vi "~POC - Video Player.vi"() -> ()   [LabVIEW 2026]
uses:
  ee0876c7-fe61-481f-ab68-a2d5c60b0e47.vi
  329ef220-7369-4e64-8ff1-382a6ca25eb8.vi
  TreeDirectoryExt/TreeDirectoryExt.lvclass
  C:/Program Files/National Instruments/LabVIEW 2026/vi.lib/QSI/QControls/QControl Classes/TreeControl/TreeControl.lvclass
panel:
  in  "Table of Contents":string(tree)
  out "Web Browser Control":string(html)
  out "Run Javascript":string
  out "Exception":string
  in  "Speed":dbl(slide)=1.0 min=0.5 max=3.0 step=0.25 scale=0.5..3.0
  in  "Checkbox":bool
  in  "Stop":bool
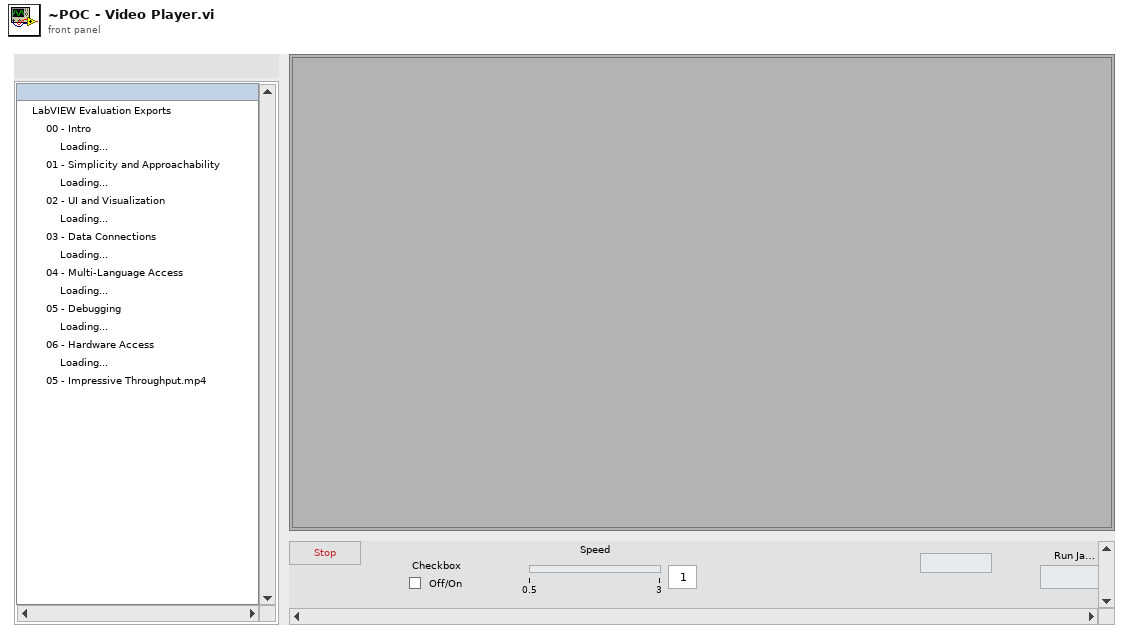
[diagram p1: front panel]
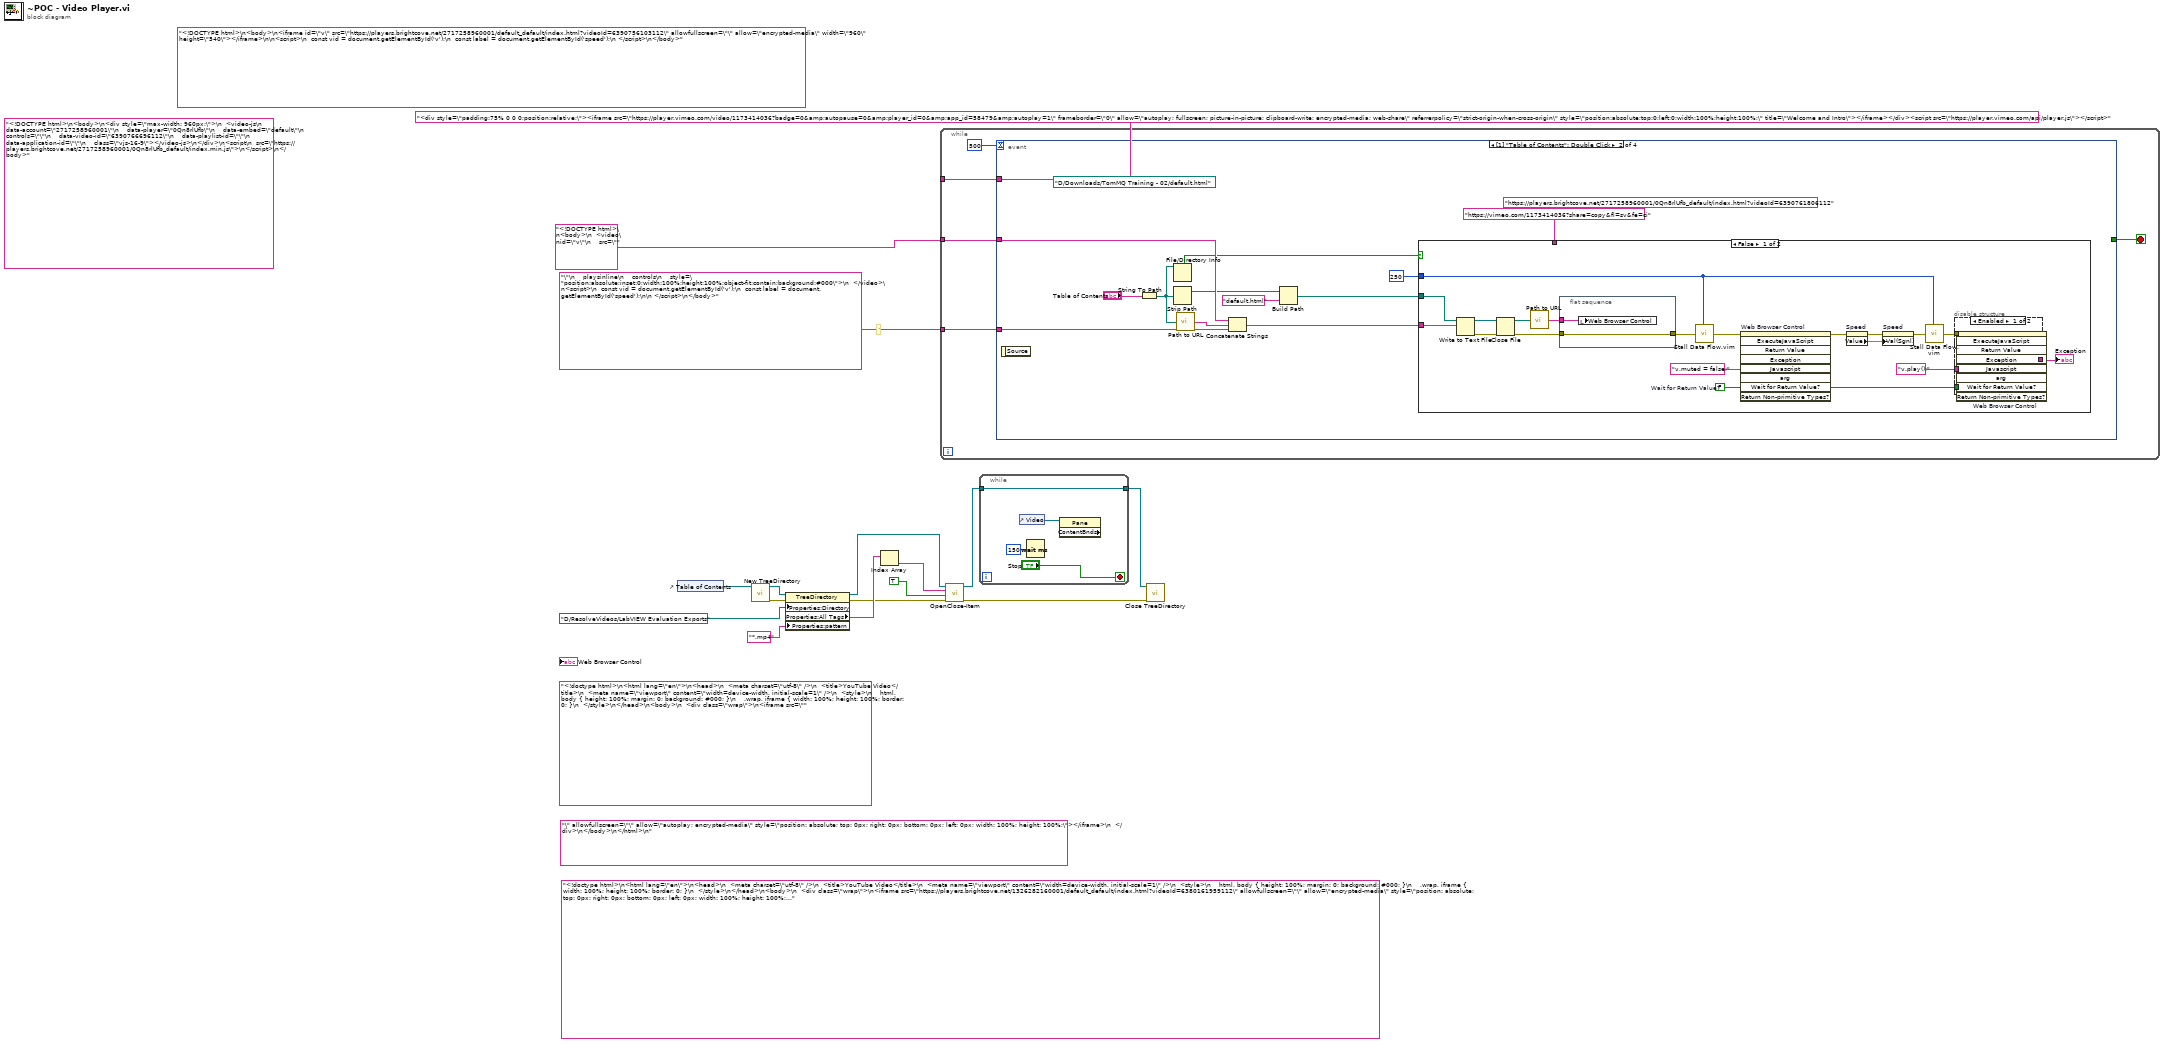
[diagram p0: block diagram]
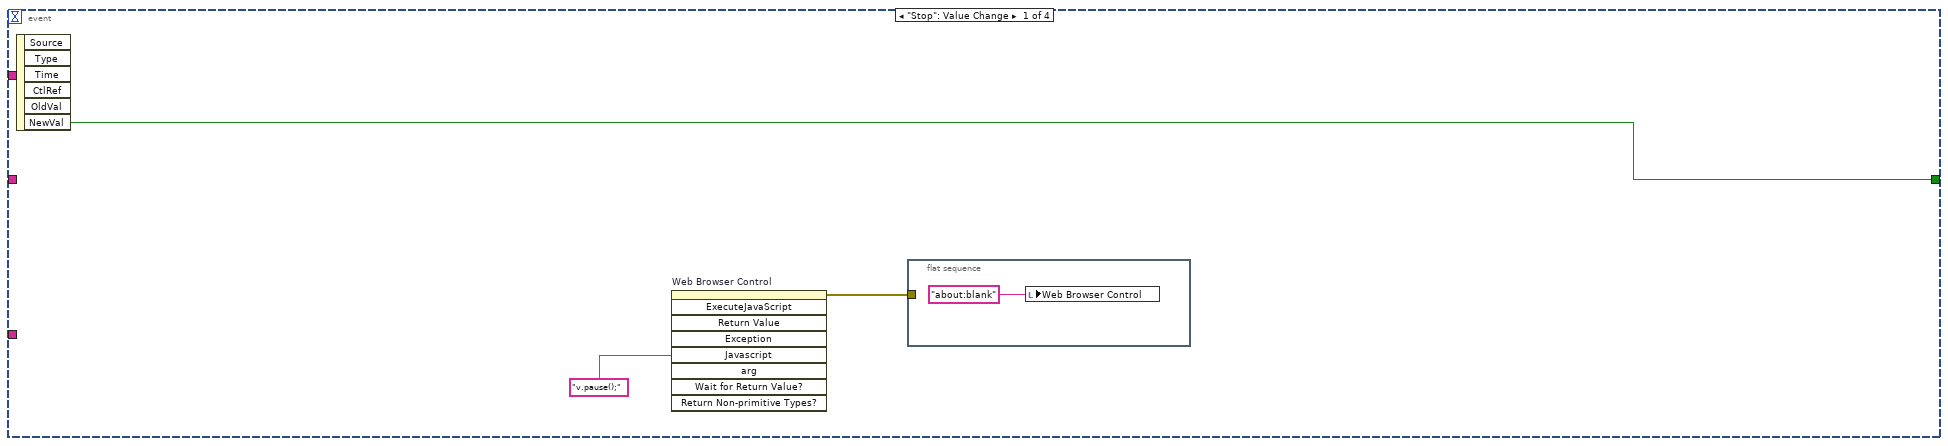
[diagram p2: hidden frame]
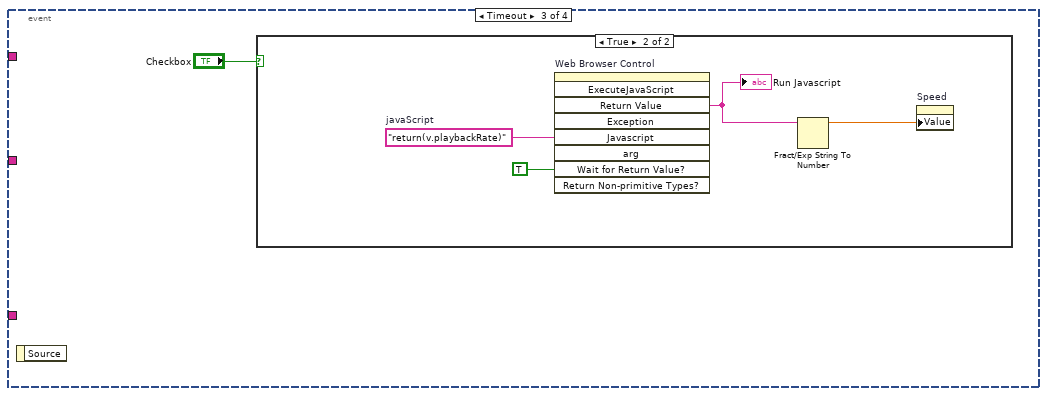
[diagram p5: hidden frame]
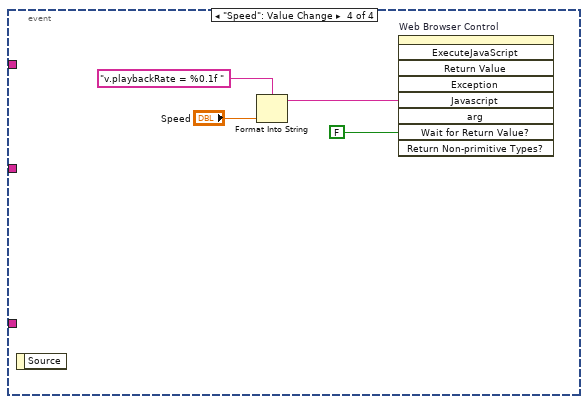
[diagram p7: hidden frame]
diagram:
  (unwired) "<!DOCTYPE html>\n<body>\n<div style=\"max-width: 960px;\">\n  <video-js\n    data-account=\"2717258960001\"\n    data-player=\"0Qn8rlUfb\"\n    data-embed=\"default\"\n    controls=\"\"\n    data-video-id=\"6390766696112\"\n    data-playlist-id=\"\"\n    data-application-id=\"\"\n    class=\"vjs-16-9\"></video-js>\n</div>\n<script\n  src=\"https://players.brightcove.net/2717258960001/0Qn8rlUfb_default/index.min.js\">\n</script>\n</body>"
  (unwired) "<!DOCTYPE html>\n<body>\n<iframe id=\"v\" src=\"https://players.brightcove.net/2717258960001/default_default/index.html?videoId=6390756103112\" allowfullscreen=\"\" allow=\"encrypted-media\" width=\"960\" height=\"540\"></iframe>\n\n<script>\n  const vid = document.getElementById('v');\n  const label = document.getElementById('speed');\n </script>\n</body>"
  (unwired) "\" allowfullscreen=\"\" allow=\"autoplay; encrypted-media\" style=\"position: absolute; top: 0px; right: 0px; bottom: 0px; left: 0px; width: 100%; height: 100%;\"></iframe>\n  </div>\n</body>\n</html>\n"
  (unwired) "<!doctype html>\n<html lang=\"en\">\n<head>\n  <meta charset=\"utf-8\" />\n  <title>YouTube Video</title>\n  <meta name=\"viewport\" content=\"width=device-width, initial-scale=1\" />\n  <style>\n    html, body { height: 100%; margin: 0; background: #000; }\n    .wrap, iframe { width: 100%; height: 100%; border: 0; }\n  </style>\n</head>\n<body>\n  <div class=\"wrap\">\n<iframe src=\"https://players.brightcove.net/1326282160001/default_default/index.html?videoId=6380161959112\" allowfullscreen=\"\" allow=\"encrypted-media\" style=\"position: absolute; top: 0px; right: 0px; bottom: 0px; left: 0px; width: 100%; height: 100%;\"></iframe>\n  </div>\n</body>\n</html>\n"
  (unwired) "<!doctype html>\n<html lang=\"en\">\n<head>\n  <meta charset=\"utf-8\" />\n  <title>YouTube Video</title>\n  <meta name=\"viewport\" content=\"width=device-width, initial-scale=1\" />\n  <style>\n    html, body { height: 100%; margin: 0; background: #000; }\n    .wrap, iframe { width: 100%; height: 100%; border: 0; }\n  </style>\n</head>\n<body>\n  <div class=\"wrap\">\n<iframe src=\""
  # "`"
  n1 = control-ref of="Table of Contents"() -> (w15:refnum<vi>)
  n2 = call "New TreeDirectory.vi"("Reference"=w15) -> ("error out"=w13:errorcluster, "TreeDirectory out"=w14:refnum<class "TreeDirectoryExt.lvclass">)  [unwired: 9 in]
  n3 = property class="TreeDirectory"(reference=w14, error in=w13, "Properties:Directory"=path "D:/ResolveVideos/LabVIEW Evaluation Exports", "Properties:pattern"="*.mp4" ("pattern")) -> (reference out=w3:refnum<class "TreeDirectoryExt.lvclass">, error out=w10:errorcluster, "Properties:All Tags"=w12:string[])
  n4 = Index Array(array=w12) -> (element=w16:string)  [unwired: 1 in]
  n5 = while {
    tunnel: "<!DOCTYPE html>\n<body>\n  <video\nid=\"v\"\n    src=\"" -> [w21]
    tunnel: "\"\n    playsinline\n    controls\n    style=\"position:absolute;inset:0;width:100%;height:100%;object-fit:contain;background:#000\">\n  </video>\n<script>\n  const vid = document.getElementById('v');\n  const label = document.getElementById('speed');\n\n </script>\n</body>" -> [w20]
    tunnel: "<div style=\"padding:75% 0 0 0;position:relative;\"><iframe src=\"https://player.vimeo.com/video/1173414036?badge=0&amp;autopause=0&amp;player_id=0&amp;app_id=58479&amp;autoplay=1\" frameborder=\"0\" allow=\"autoplay; fullscreen; picture-in-picture; clipboard-write; encrypted-media; web-share\" referrerpolicy=\"strict-origin-when-cross-origin\" style=\"position:absolute;top:0;left:0;width:100%;height:100%;\" title=\"Welcome and Intro\"></iframe></div><script src=\"https://player.vimeo.com/api/player.js\"></script>" -> [w17]
    stop <- w19 stop-if-true
    n6 = event shown="[1] \"Table of Contents\": Double Click" {
      selector: _ -> [_ _ _ _]
      dyn-events: _ -> [_ _ _ _]
      timeout: 500 -> [_ _ _ _]
      tunnel: w21 -> [_ w36 _ _]
      tunnel: w20 -> [_ w35 _ _]
      tunnel: [w24 _ _ _] -> w19
      tunnel: w17 -> [_ _ _ _]
      event "Stop": Value Change {
        n7 = event-data() -> ("NewVal"=w24:bool)  [unwired: 1 in, 5 out]
        n8 = invoke on="Web Browser Control" class="WebBrowser (strict)" method="ExecuteJavaScript"("Javascript"="v.pause();" ("javaScript")) -> (error out=w22:errorcluster)  [unwired: 8 in, 8 out]
        n9 = flat-sequence {
          tunnel: w22 -> [_]
          frame #0 {
            n10 = local write "Web Browser Control"("about:blank") -> ()
          }
        }
      }
      event "Table of Contents": Double Click {
        (unwired) "https://players.brightcove.net/2717258960001/0Qn8rlUfb_default/index.html?videoId=6390761806112"
        (unwired) path "D:/Downloads/TomMQ Training - 02/default.html"
        n11 = event-data() -> ()  [unwired: 1 in, 1 out]
        n12 = String To Path(string="Table of Contents") -> (path=w29:path)
        n13 = File/Directory Info(path=w29) -> (directory=w30:bool)  [unwired: 1 in, 6 out]
        n14 = Strip Path(path=w29) -> (stripped path=w33:path)  [unwired: 1 out]
        n15 = call <vilib>:"Path to URL.vi"("path"=w29) -> ("url"=w28:string)
        n16 = Concatenate Strings(w36, w28, w35) -> (w26:string)
        n17 = Build Path(base path=w33, name or relative path="default.html") -> (appended path=w32:path)
        n18 = case shown="False" w30 {
          tunnel: w32 -> [w56 _]
          tunnel: w26 -> [w55 _]
          tunnel: u32 250 ("milliseconds to wait") -> [w43 _]
          tunnel: "https://vimeo.com/1173414036?share=copy&fl=sv&fe=ci" -> [_ _]
          frame False {
            w42 = FALSE  # Wait for Return Value?
            n19 = Write to Text File(file (use dialog)=w56, text=w55) -> (refnum out=w53:refnum<file>, error out=w54:errorcluster)  [unwired: 2 in, 1 out]
            n20 = Close File(refnum=w53, error in=w54) -> (path=w46:path, error out=w49:errorcluster)
            n21 = call <vilib>:"Path to URL.vi"("path"=w46) -> ("url"=w38:string)
            n22 = flat-sequence {
              tunnel: [w63] -> w50
              tunnel: w49 -> [w63]
              tunnel: w38 -> [w62]
              frame #0 {
                n23 = local write "Web Browser Control"(w62) -> ()
              }
            }
            n24 = call "Stall Data Flow.vim"("value in"=w50, "milliseconds to wait"=w43) -> ("value out"=w40:errorcluster)  [unwired: 1 out]
            n25 = invoke on="Web Browser Control" class="WebBrowser (strict)" method="ExecuteJavaScript"(error in=w40, "Javascript"="v.muted = false;" ("javaScript"), "Wait for Return Value?"=w42) -> (error out=w47:errorcluster)  [unwired: 6 in, 8 out]
            n26 = property on="Speed" class="Slide (strict)"(error in=w47) -> (error out=w51:errorcluster, "Value"=w52:dbl)  [unwired: 1 in, 1 out]
            n27 = property on="Speed" class="Slide (strict)"(error in=w51, "Val(Sgnl)"=w52) -> (error out=w45:errorcluster)  [unwired: 1 in, 1 out]
            n28 = call "Stall Data Flow.vim"("value in"=w45, "milliseconds to wait"=w43) -> ("value out"=w39:errorcluster)  [unwired: 1 out]
            n29 = disable-structure shown="Enabled" {
              disable-tunnel: "v.play();" ("javaScript") -> [w60 w61]
              disable-tunnel: w42 -> [w59 _]
              disable-tunnel: [w58 w61] -> w41
              disable-tunnel: w39 -> [w57 _]
              frame Enabled {
                n30 = invoke on="Web Browser Control" class="WebBrowser (strict)" method="ExecuteJavaScript"(error in=w57, "Javascript"=w60, "Wait for Return Value?"=w59) -> ("Exception"=w58:string)  [unwired: 6 in, 8 out]
              }
              frame Disabled {
              }
            }
            "Exception" <- w41
          }
          frame True {
          }
        }
      }
      event Timeout {
        n31 = event-data() -> ()  [unwired: 1 in, 1 out]
        n32 = case shown="True" "Checkbox" {
          frame False {
          }
          frame True {
            w67 = "return(v.playbackRate)"  # javaScript
            n33 = invoke on="Web Browser Control" class="WebBrowser (strict)" method="ExecuteJavaScript"("Javascript"=w67, "Wait for Return Value?"=TRUE ("Fetch Result")) -> ("Return Value"=w65:string)  [unwired: 7 in, 8 out]
            "Run Javascript" <- w65
            n34 = Fract/Exp String To Number(string=w65) -> (number=w66:dbl)  [unwired: 3 in, 1 out]
            n35 = property on="Speed" class="Slide (strict)"("Value"=w66) -> ()  [unwired: 2 in, 2 out]
          }
        }
      }
      event "Speed": Value Change {
        n36 = event-data() -> ()  [unwired: 1 in, 1 out]
        n37 = Format Into String(format string="v.playbackRate = %0.1f " ("javaScript"), "Speed") -> (resulting string=w70:string)  [unwired: 2 in, 1 out]
        n38 = invoke on="Web Browser Control" class="WebBrowser (strict)" method="ExecuteJavaScript"("Javascript"=w70, "Wait for Return Value?"=FALSE ("Decode Result")) -> ()  [unwired: 7 in, 9 out]
      }
    }
  }
  n39 = call-dynamic "OpenClose-Item.vi"("error in (no error)"=w10, "Open?"=TRUE, "Tag"=w16, "TreeDirectoryExt in"=w3) -> ("error out"=w7:errorcluster, "TreeDirectoryExt out"=w9:refnum<class "TreeDirectoryExt.lvclass">)  [unwired: 6 in]
  n40 = while {
    tunnel: w9 -> [w73]
    tunnel: [w73] -> w8
    stop <- "Stop" stop-if-true
    n41 = control-ref of="Video"() -> (w74:refnum<vi>)
    n42 = Wait (ms)(milliseconds to wait=u32 150) -> ()  [unwired: 1 out]
    n43 = property class="Pane" props=["ContentBnds"](reference=w74) -> ()  [unwired: 1 in, 3 out]
  }
  n44 = call "Close TreeDirectory.vi"("error in (no error)"=w7, "TreeDirectory in"=w8) -> ()  [unwired: 8 in, 2 out]
